vi "dfd_Convert INT Coefficients to String.vi"(5 "indent order":i32, 6 "Gain on Target?":bool, 7 "type":T1, 8 "quantized 1":i32, 9 "int gain":cluster{"wl":i16, "integer":i32}, 10 "int coef a":cluster{"wl":i16, "integers":i32[]}, 11 "int coef b":cluster{"wl":i16, "integers":i32[]}) -> (3 "xml string out":string)   [LabVIEW 2017, in "NI_DigFilter_Process.lvlib"]
uses:
  <vilib>/addons/Digital Filter Design/NI_DigFilter_Process.lvlib
  <vilib>/addons/Digital Filter Design/_Objects.llb/DFD Filter Structure Type Selector.ctl
  <vilib>/addons/Digital Filter Design/NI_DigFilterLicensed.lvlib
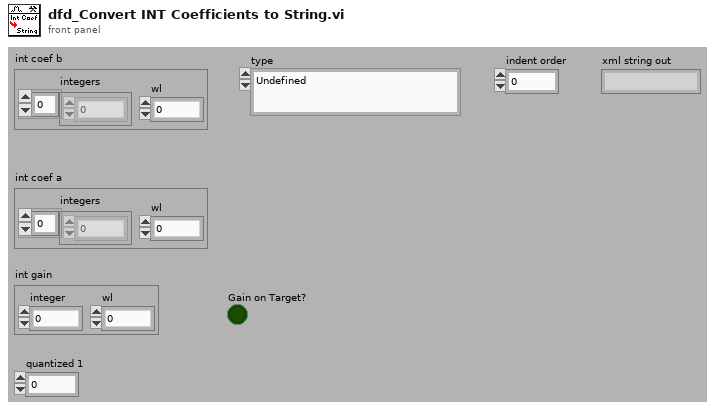
[diagram p1: front panel]
types:
  T1 = typedef "NI_DigFilterLicensed.lvlib/DFD Filter Structure Type Selector.ctl" = enum16{"Undefined", "FIR Direct Form", "FIR Direct Form Transposed", "FIR Symmetric", "FIR Antisymmetric", "IIR Direct Form I", "IIR Direct Form I Transposed", "IIR Direct Form II", "IIR Direct Form II Transposed", "IIR Cascaded Second Order Sections Form I", "IIR Cascaded Second Order Sections Form I Transposed", "IIR Cascaded Second Order Sections Form II", "IIR Cascaded Second Order Sections Form II Transposed", "Lattice Allpass (basic sections)", "Lattice Allpass (one multiplier sections)", "Lattice Allpass (normalized sections)", "Lattice AR (basic sections)", "Lattice AR (one multiplier sections)", "Lattice AR (normalized sections)", "Lattice MA (minimum phase)", "Lattice MA (maximum phase)", "Lattice ARMA (basic sections)", "Lattice ARMA (one multiplier sections)", "Lattice ARMA (normalized sections)"}
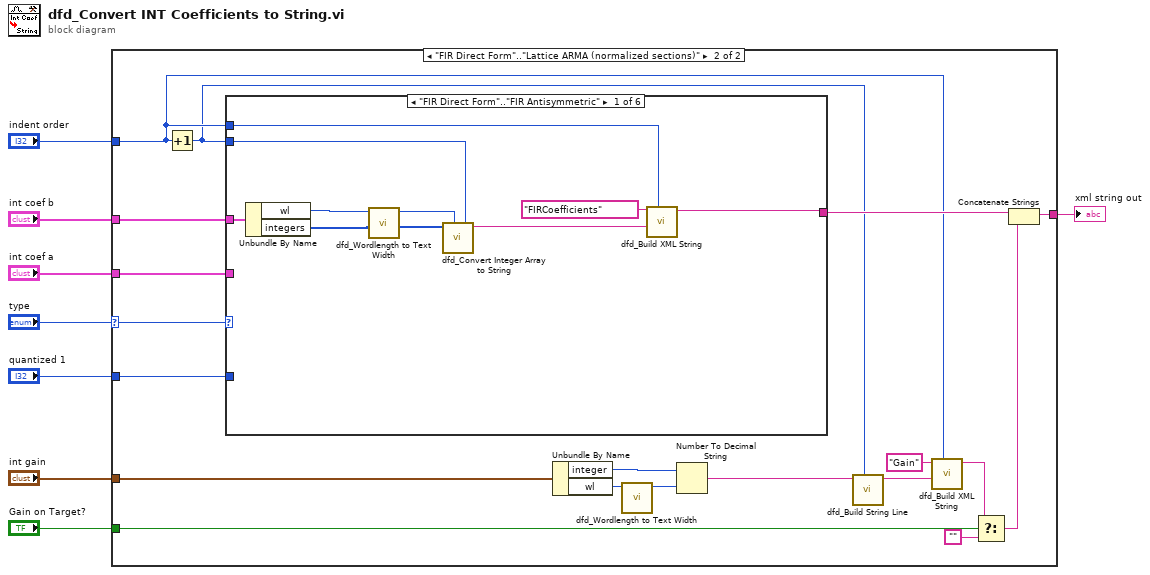
[diagram p0: block diagram]
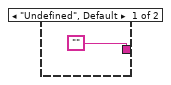
[diagram p2: hidden frame]
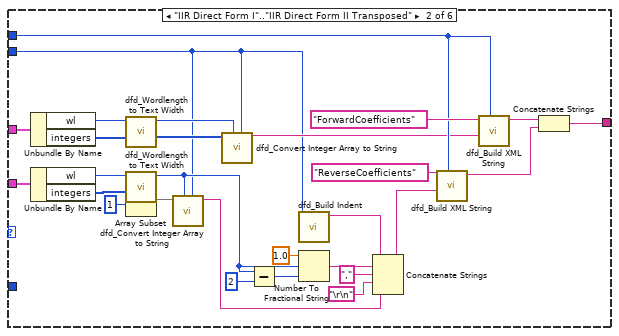
[diagram p3: hidden frame]
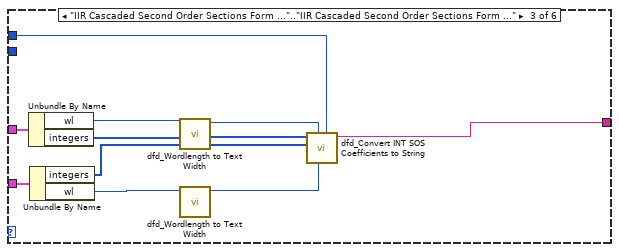
[diagram p4: hidden frame]
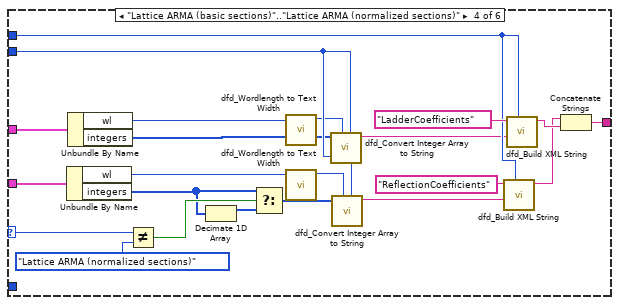
[diagram p5: hidden frame]
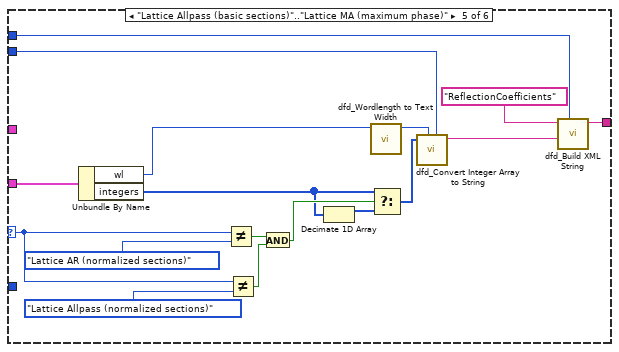
[diagram p6: hidden frame]
diagram:
  n1 = case shown="\"FIR Direct Form\"..\"Lattice ARMA (normalized sections)\"" "type" {
    selector: "type" -> [_ w23]
    tunnel: ["" w26] -> w8
    tunnel: "indent order" -> [_ w25]
    tunnel: "int coef b" -> [_ w22]
    tunnel: "int coef a" -> [_ w21]
    tunnel: "int gain" -> [_ w20]
    tunnel: "quantized 1" -> [_ w16]
    tunnel: "Gain on Target?" -> [_ w15]
    frame "Undefined", Default {
    }
    frame "FIR Direct Form".."Lattice ARMA (normalized sections)" {
      n2 = Increment(x=w25) -> (x+1=w24:i32)
      n3 = case shown="\"FIR Direct Form\"..\"FIR Antisymmetric\"" w23 {
        selector: w23 -> [_ _ _ w82 w106 _]
        tunnel: [w36 w59 w73 w93 w111 _] -> w27
        tunnel: w25 -> [w35 w62 w74 w94 w112 _]
        tunnel: w24 -> [w33 w40 _ w90 w109 _]
        tunnel: w22 -> [w32 w55 w72 w87 _ _]
        tunnel: w21 -> [_ w53 w68 w81 w108 _]
        tunnel: w16 -> [_ _ _ _ _ _]
        frame "FIR Direct Form".."FIR Antisymmetric" {
          n4 = Unbundle By Name(w32) -> ("wl"=w31:i16, "integers"=w29:i32[])
          n5 = call <vilib>:"dfd_Wordlength to Text Width.vi"("wl"=w31) -> ("width"=w30:i16)  [unwired: 1 in, 9 out]
          n6 = call <vilib>:"dfd_Convert Integer Array to String.vi"("indent order"=w33, "width (-)"=w30, "I32 values"=w29) -> ("string"=w34:string)  [unwired: 2 in, 6 out]
          n7 = call <vilib>:"dfd_Build XML String.vi"("indent order"=w35, "string in"=w34, "element name"="FIRCoefficients") -> ("xml string out"=w36:string)  [unwired: 1 in, 7 out]
        }
        frame "IIR Direct Form I".."IIR Direct Form II Transposed" {
          n8 = Unbundle By Name(w55) -> ("wl"=w57:i16, "integers"=w54:i32[])
          n9 = Unbundle By Name(w53) -> ("wl"=w52:i16, "integers"=w43:i32[])
          n10 = call <vilib>:"dfd_Wordlength to Text Width.vi"("wl"=w57) -> ("width"=w56:i16)  [unwired: 1 in, 9 out]
          n11 = call <vilib>:"dfd_Wordlength to Text Width.vi"("wl"=w52) -> ("width"=w45:i16)  [unwired: 1 in, 9 out]
          n12 = Array Subset(array=w43, index=1) -> (w42:i32[])  [unwired: 1 in]
          n13 = call <vilib>:"dfd_Convert Integer Array to String.vi"("indent order"=w40, "width (-)"=w45, "I32 values"=w42) -> ("string"=w39:string)  [unwired: 2 in, 6 out]
          n14 = call <vilib>:"dfd_Convert Integer Array to String.vi"("indent order"=w40, "width (-)"=w56, "I32 values"=w54) -> ("string"=w58:string)  [unwired: 2 in, 6 out]
          n15 = Subtract(x=w45, y=i16 2) -> (x-y=w50:i16)
          n16 = call <vilib>:"dfd_Build Indent.vi"("indent order"=w40) -> ("tag indent"=w46:string)  [unwired: 10 out]
          n17 = Number To Fractional String(number=1.0, width (-)=w45, precision (6)=w50) -> (F-format string=w47:string)  [unwired: 1 out]
          n18 = Concatenate Strings(w46, w47, "," ("string"), "\r\n", w39) -> (w44:string)
          n19 = call <vilib>:"dfd_Build XML String.vi"("indent order"=w62, "string in"=w44, "element name"="ReverseCoefficients") -> ("xml string out"=w60:string)  [unwired: 1 in, 7 out]
          n20 = call <vilib>:"dfd_Build XML String.vi"("indent order"=w62, "string in"=w58, "element name"="ForwardCoefficients") -> ("xml string out"=w61:string)  [unwired: 1 in, 7 out]
          n21 = Concatenate Strings(w61, w60) -> (w59:string)
        }
        frame "IIR Cascaded Second Order Sections Form I".."IIR Cascaded Second Order Sections Form II Transposed" {
          n22 = Unbundle By Name(w72) -> ("wl"=w71:i16, "integers"=w69:i32[])
          n23 = Unbundle By Name(w68) -> ("integers"=w65:i32[], "wl"=w67:i16)
          n24 = call <vilib>:"dfd_Wordlength to Text Width.vi"("wl"=w71) -> ("width"=w70:i16)  [unwired: 1 in, 9 out]
          n25 = call <vilib>:"dfd_Wordlength to Text Width.vi"("wl"=w67) -> ("width"=w66:i16)  [unwired: 1 in, 9 out]
          n26 = call <vilib>:"dfd_Convert INT SOS Coefficients to String.vi"("indent order"=w74, "width (a)"=w66, "width (b)"=w70, "coef a"=w65, "coef b"=w69) -> ("XML string out"=w73:string)  [unwired: 1 in, 5 out]
        }
        frame "Lattice ARMA (basic sections)".."Lattice ARMA (normalized sections)" {
          n27 = Unbundle By Name(w81) -> ("wl"=w80:i16, "integers"=w78:i32[])
          n28 = Unbundle By Name(w87) -> ("wl"=w85:i16, "integers"=w86:i32[])
          n29 = Not Equal?(x=w82, y=DFD_Filter_Structure_Type_Selector."Lattice ARMA (normalized sections)" ("type 2")) -> (x != y?=w89:bool)
          n30 = Decimate 1D Array(w78) -> (w88:i32[])  [unwired: 1 out]
          n31 = Select(t=w78, s=w89, f=w88) -> (s? t:f=w77:i32[])
          n32 = call <vilib>:"dfd_Wordlength to Text Width.vi"("wl"=w85) -> ("width"=w84:i16)  [unwired: 1 in, 9 out]
          n33 = call <vilib>:"dfd_Wordlength to Text Width.vi"("wl"=w80) -> ("width"=w79:i16)  [unwired: 1 in, 9 out]
          n34 = call <vilib>:"dfd_Convert Integer Array to String.vi"("indent order"=w90, "width (-)"=w84, "I32 values"=w86) -> ("string"=w92:string)  [unwired: 2 in, 6 out]
          n35 = call <vilib>:"dfd_Convert Integer Array to String.vi"("indent order"=w90, "width (-)"=w79, "I32 values"=w77) -> ("string"=w91:string)  [unwired: 2 in, 6 out]
          n36 = call <vilib>:"dfd_Build XML String.vi"("indent order"=w94, "string in"=w91, "element name"="ReflectionCoefficients") -> ("xml string out"=w75:string)  [unwired: 1 in, 7 out]
          n37 = call <vilib>:"dfd_Build XML String.vi"("indent order"=w94, "string in"=w92, "element name"="LadderCoefficients") -> ("xml string out"=w76:string)  [unwired: 1 in, 7 out]
          n38 = Concatenate Strings(w75, w76) -> (w93:string)
        }
        frame "Lattice Allpass (basic sections)".."Lattice MA (maximum phase)" {
          n39 = Unbundle By Name(w108) -> ("wl"=w98:i16, "integers"=w100:i32[])
          n40 = Not Equal?(x=w106, y=DFD_Filter_Structure_Type_Selector."Lattice AR (normalized sections)" ("type 2")) -> (x != y?=w104:bool)
          n41 = Not Equal?(x=w106, y=DFD_Filter_Structure_Type_Selector."Lattice Allpass (normalized sections)" ("type 2")) -> (x != y?=w103:bool)
          n42 = And(x=w104, y=w103) -> (x .and. y?=w101:bool)
          n43 = Decimate 1D Array(w100) -> (w102:i32[])  [unwired: 1 out]
          n44 = call <vilib>:"dfd_Wordlength to Text Width.vi"("wl"=w98) -> ("width"=w97:i16)  [unwired: 1 in, 9 out]
          n45 = Select(t=w100, s=w101, f=w102) -> (s? t:f=w99:i32[])
          n46 = call <vilib>:"dfd_Convert Integer Array to String.vi"("indent order"=w109, "width (-)"=w97, "I32 values"=w99) -> ("string"=w110:string)  [unwired: 2 in, 6 out]
          n47 = call <vilib>:"dfd_Build XML String.vi"("indent order"=w112, "string in"=w110, "element name"="ReflectionCoefficients") -> ("xml string out"=w111:string)  [unwired: 1 in, 7 out]
        }
        frame Default {
        }
      }
      n48 = Unbundle By Name(w20) -> ("integer"=w17:i32, "wl"=w19:i16)
      n49 = call <vilib>:"dfd_Wordlength to Text Width.vi"("wl"=w19) -> ("width"=w18:i16)  [unwired: 1 in, 9 out]
      n50 = Number To Decimal String(number=w17, width (-)=w18) -> (decimal integer string=w12:string)
      n51 = call <vilib>:"dfd_Build String Line.vi"("indent order"=w24, "string"=w12) -> ("string line"=w13:string)  [unwired: 9 out]
      n52 = call <vilib>:"dfd_Build XML String.vi"("indent order"=w25, "string in"=w13, "element name"="Gain") -> ("xml string out"=w11:string)  [unwired: 1 in, 7 out]
      n53 = Select(t=w11, s=w15, f="") -> (s? t:f=w10:string)
      n54 = Concatenate Strings(w27, w10) -> (w26:string)
    }
  }
  "xml string out" <- w8
